vi "formatTrac.vi"(7 "Channel":bool, 8 "error in (no error)":errorcluster, 9 "Temperature":bool, 10 "Timestamp":bool, 11 "Electrometer in":refnum<class "Electrometer.lvclass">) -> (0 "error out":errorcluster, 2 "command":string, 3 "Electrometer out":refnum<class "Electrometer.lvclass">)   [LabVIEW 2016, in "Electrometer.lvclass"]
uses:
  Electrometer.lvclass
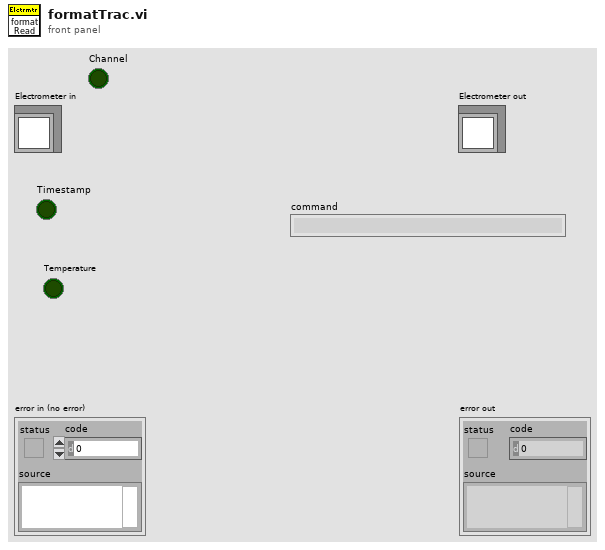
[diagram p1: front panel]
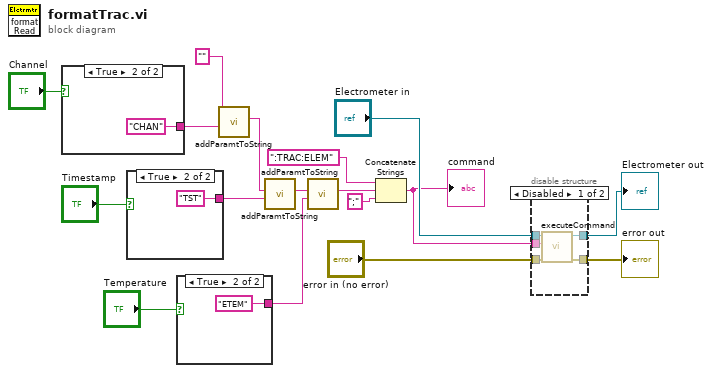
[diagram p0: block diagram]
diagram:
  n1 = case shown="True" "Channel" {
    tunnel: [_ "CHAN" ("command")] -> w7
    frame False {
    }
    frame True {
    }
  }
  n2 = case shown="True" "Timestamp" {
    tunnel: [_ "TST" ("command")] -> w5
    frame False {
    }
    frame True {
    }
  }
  n3 = case shown="True" "Temperature" {
    tunnel: [_ "ETEM" ("command")] -> w3
    frame False {
    }
    frame True {
    }
  }
  n4 = call "addParamtToString.vi"("param"=w7, "paramList in"="") -> ("paramList out"=w6:string)  [unwired: 7 in, 2 out]
  n5 = call "addParamtToString.vi"("param"=w5, "paramList in"=w6) -> ("paramList out"=w4:string)  [unwired: 7 in, 2 out]
  n6 = call "addParamtToString.vi"("param"=w3, "paramList in"=w4) -> ("paramList out"=w2:string)  [unwired: 7 in, 2 out]
  n7 = Concatenate Strings(":TRAC:ELEM" ("command"), w2, ";" ("string")) -> (w13:string)
  "command" <- w13
  n8 = disable-structure shown="Disabled" {
    disable-tunnel: "Electrometer in" -> [w25 _]
    disable-tunnel: [w24 _] -> w16
    disable-tunnel: [w23 _] -> w15
    disable-tunnel: "error in (no error)" -> [w22 _]
    disable-tunnel: w13 -> [w21 _]
    frame Disabled {
      n9 = call "executeCommand.vi"("error in (no error)"=w22, "command"=w21, "Electrometer in"=w25) -> ("error out"=w23:errorcluster, "Electrometer out"=w24:refnum<class "Electrometer.lvclass">)  [unwired: 7 in]
    }
    frame Enabled {
    }
  }
  "error out" <- w15
  "Electrometer out" <- w16
